vi "Build State String with Arguments__JKI_lib_State_Machine.vi"(4 "Arguments (\"\")":string, 5 "State":string) -> (1 "State with Arguments":string)   [LabVIEW 2020]
doc: "Builds a state string that contains arguments for the JKI State Machine.\n<B>For Example:</B> If State = A and Arguments = B then State with Arguments = A >> B\n\nFor instructions on how to use the JKI State Machine, examples and video tutorials, visit:\nhttp://jkisoft.com/state-machine/\n\n<B>Inputs:</B>\n <B>State:</B> The State string that requires the argument.\n <B>Arguments:</B> The Argument string to add to the state. The default is an empty string. If Argument is an empty string then State will be returned to the output. <B>Note:</B> The arguments input must not contain any unprintable characters like linefeed or carriage return.\n\n<B>Outputs:</B>\n <B>State with Arguments:</B> This output returns the new string that contains the State and the Argument. <B>For Example:</B> If State = A and Arguments = B then State with Arguments = A >> B\n\nJKI State Machine™ 2018.0.7.45\nhttp://jki.net/state-machine/\nCopyright (C) 2005-2018, JKI <info@jki.net>\nALL RIGHTS RESERVED"
panel:
  # "For instructions on how to use the JKI State Machine, examples and video tutorials, visit:\nhttp://jki.net/state-machine/\n\nJKI State Machine™\nhttp://jki.net/state-machine/\nCopyright (C) 2005-2017, JKI <info@jki.net>\nALL RIGHTS RESERVED"
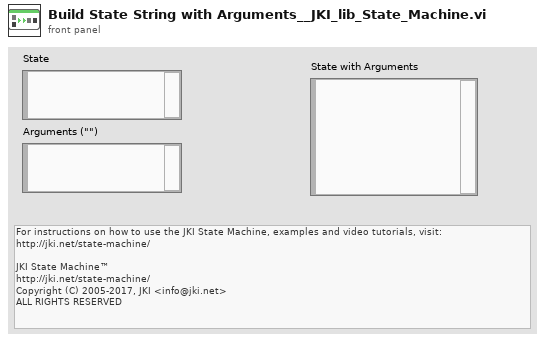
[diagram p1: front panel]
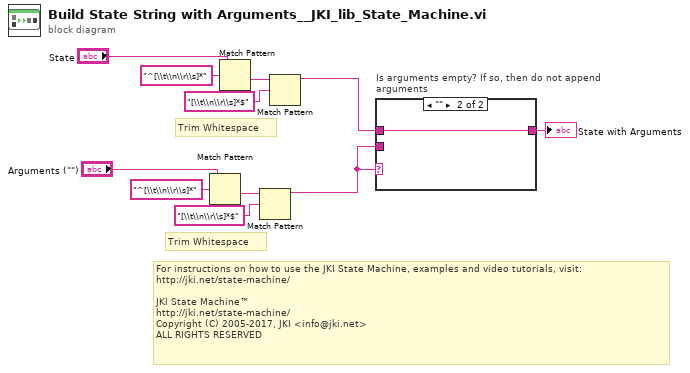
[diagram p0: block diagram]
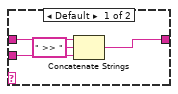
[diagram p2: hidden frame]
diagram:
  # "For instructions on how to use the JKI State Machine, examples and video tutorials, visit:\nhttp://jki.net/state-machine/\n\nJKI State Machine™\nhttp://jki.net/state-machine/\nCopyright (C) 2005-2017, JKI <info@jki.net>\nALL RIGHTS RESERVED"
  # "Trim Whitespace"
  # "Trim Whitespace"
  n1 = Match Pattern(string="Arguments (\"\")", regular expression="^[\\t\\n\\r\\s]*") -> (after substring=w4:string)  [unwired: 1 in, 3 out]
  n2 = Match Pattern(string="State", regular expression="^[\\t\\n\\r\\s]*") -> (after substring=w9:string)  [unwired: 1 in, 3 out]
  n3 = Match Pattern(string=w4, regular expression="[\\t\\n\\r\\s]*$") -> (before substring=w1:string)  [unwired: 1 in, 3 out]
  n4 = Match Pattern(string=w9, regular expression="[\\t\\n\\r\\s]*$") -> (before substring=w6:string)  [unwired: 1 in, 3 out]
  n5 = case "Is arguments empty? If so, then do not append arguments" shown="\"\"" w1 {
    tunnel: [w12 w16] -> w11
    tunnel: w6 -> [w15 w16]
    tunnel: w1 -> [w13 _]
    frame Default {
      n6 = Concatenate Strings(w15, " >> " ("string"), w13) -> (w12:string)
    }
    frame "" {
    }
  }
  "State with Arguments" <- w11
